vi "Get lastsettings.vi"(4 "error in":errorcluster) -> (0 "error out":errorcluster, 2 "VNALogOpt":T1={"VNALogSelect"=enum."No Selection", "VNALogTIncr"=5.0, "VNALogTList"=""} caption="VNA Log Option" {"VNALogTIncr" min=1.0 step=1.0 format="%#.1g"}, 3 "Path":path)   [LabVIEW 2023]
uses:
  controls/VNALogOpt.ctl
  <vilib>/Utility/sysdir.llb/System Directory Type.ctl
  <vilib>/Utility/config.llb/Read Key (Path).vi
  <vilib>/Utility/config.llb/Write Key (Path).vi
  <vilib>/Utility/config.llb/NI_LVConfig.lvlib
  <userlib>/_OpenG.lib/variantconfig/variantconfig.llb/openg_variant_configuration_file.lvlib
panel:
  out "appended path":path
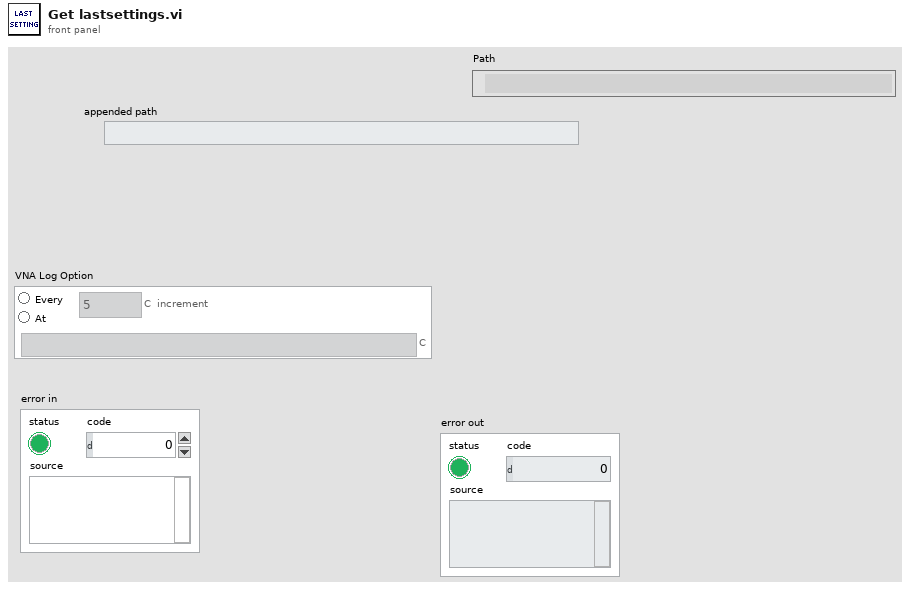
[diagram p1: front panel]
types:
  T1 = typedef "VNALogOpt.ctl" = cluster{"VNALogSelect":enum32{"No Selection", "TempIncr", "TempList"}, "VNALogTIncr":dbl, "VNALogTList":string}
  T2 = typedef "NI_LVConfig.lvlib/Config Data RefNum.ctl" = refnum<k1>
  T3 = typedef "System Directory Type.ctl" = i32
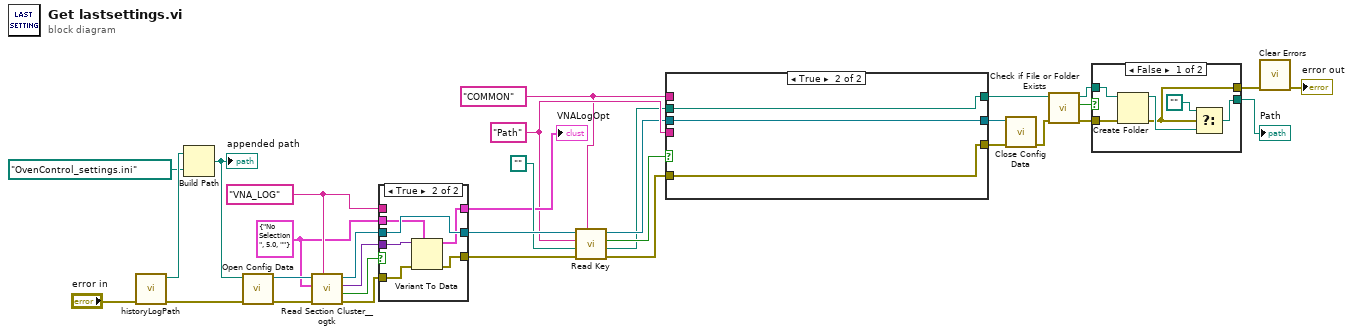
[diagram p0: block diagram]
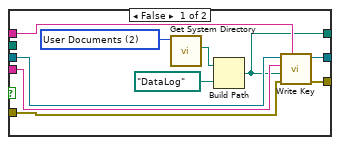
[diagram p3: hidden frame]
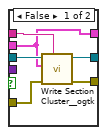
[diagram p4: hidden frame]
diagram:
  w16 = "Path" ("key")
  w15 = "COMMON" ("section")
  w25 = "VNA_LOG" ("section (optional)")
  w23 = T1 {"VNALogSelect"=enum."No Selection", "VNALogTIncr"=5.0, "VNALogTList"=""} ("VNALogOpt")
  n1 = call "historyLogPath.vi"("error in"="error in") -> ("error out"=w30:errorcluster, "Path Out"=w33:path)  [unwired: 4 in, 1 out]
  n2 = Build Path(base path=w33, name or relative path=path "OvenControl_settings.ini") -> (appended path=w31:path)
  "appended path" <- w31
  n3 = call <vilib>:"Open Config Data.vi"("error in (no error)"=w30, "configuration file path"=w31) -> ("error out"=w28:errorcluster, "refnum"=w29:T2)  [unwired: 7 in, 1 out]
  n4 = call <userlib>:"Read Section Cluster__ogtk.vi"("section (optional)"=w25, "error in (no error)"=w28, "Section Formatted Cluster Type"=w23, "refnum"=w29) -> ("error out"=w24:errorcluster, "all found?"=w27:bool, "Section Formatted Cluster"=w19:variant, "dup refnum"=w26:T2)  [unwired: 3 in, 1 out]
  n5 = case shown="True" w27 {
    tunnel: w26 -> [w39 w45]
    tunnel: w25 -> [w38 _]
    tunnel: w24 -> [w37 w41]
    tunnel: w23 -> [w34 w43]
    tunnel: [w36 w45] -> w22
    tunnel: [w35 w40] -> w20
    tunnel: [w34 w42] -> w18
    tunnel: w19 -> [_ w44]
    frame False {
      n6 = call <userlib>:"Write Section Cluster__ogtk.vi"("section (optional)"=w38, "error in (no error)"=w37, "Section Formatted Cluster"=w34, "refnum"=w39) -> ("error out"=w35:errorcluster, "dup refnum"=w36:T2)  [unwired: 6 in]
    }
    frame True {
      n7 = Variant To Data(error in=w41, type=w43, Variant=w44) -> (data=w42:T1, error out=w40:errorcluster)
    }
  }
  "VNALogOpt" <- w18
  n8 = call-poly <vilib>:"Read Key.vi"("section"=w15, "error in (no error)"=w20, "default value"=path "", "key"=w16, "refnum"=w22) -> ("error out"=w13:errorcluster, "value"=w10:path, "found?"=w17:bool, "refnum out"=w14:T2)  [unwired: 3 in]
  n9 = case shown="True" w17 {
    tunnel: w16 -> [w52 _]
    tunnel: w15 -> [w51 _]
    tunnel: w14 -> [w50 w57]
    tunnel: w13 -> [w49 w58]
    tunnel: [w48 w57] -> w12
    tunnel: [w47 w58] -> w11
    tunnel: [w46 w56] -> w9
    tunnel: w10 -> [_ w56]
    frame False {
      w55 = T3 2 items=["User Home"=0, "User Desktop"=1, "User Documents"=2, "User Application Data"=3, "User Preferences"=4, "User Temporary"=5, "Public Documents"=6, "Public Application Data"=7, "Public Preferences"=8, "Public Cache"=13, "System Core Libraries"=9, "System Installed Libraries"=10, "Application Files"=11, "Boot Volume Root"=12] ("system directory type")
      n10 = call <vilib>:"Get System Directory.vi"("system directory type"=w55) -> ("system directory"=w54:path)  [unwired: 10 in]
      n11 = Build Path(base path=w54, name or relative path=path "DataLog") -> (appended path=w46:path)
      n12 = call-poly <vilib>:"Write Key.vi"("section"=w51, "error in (no error)"=w49, "value"=w46, "key"=w52, "refnum"=w50) -> ("error out"=w47:errorcluster, "refnum out"=w48:T2)  [unwired: 4 in, 1 out]
    }
    frame True {
    }
  }
  n13 = call <vilib>:"Close Config Data.vi"("error in (no error)"=w11, "refnum"=w12) -> ("error out"=w8:errorcluster)  [unwired: 8 in, 1 out]
  n14 = call <vilib>:"Check if File or Folder Exists.vi"("error in (no error)"=w8, "path"=w9) -> ("error out"=w5:errorcluster, "file or folder exists?"=w7:bool, "dup path"=w6:path)  [unwired: 7 in]
  n15 = case shown="False" w7 {
    tunnel: w6 -> [w64 w66]
    tunnel: w5 -> [w63 w65]
    tunnel: [w60 w66] -> w4
    tunnel: [w59 w65] -> w3
    frame False {
      n16 = Create Folder(path (use dialog)=w64, error in=w63) -> (created path=w62:path, error out=w59:errorcluster)  [unwired: 1 in, 1 out]
      n17 = Select(t=path "", s=w59, f=w62) -> (s? t:f=w60:path)
    }
    frame True {
    }
  }
  "Path" <- w4
  n18 = call <vilib>:"Clear Errors.vi"("error in (no error)"=w3) -> ("error out"=→"error out":errorcluster)  [unwired: 5 in, 1 out]
